vi "MT Generate PAM system parameters (M).vi"(0 "samples per symbol (16)":i32=16, 5 "M-PAM (2)":i32=2, 11 "error in (no error)":errorcluster) -> (6 "PAM system parameters":T1 {"symbol map" format="%.3f"}, 8 "bits per symbol":i32, 15 "error out":errorcluster)   [LabVIEW 2020, in "niDMT.lvlib"]
doc: "This polymorphic instance calculates parameters for use with either the MT Modulate PAM VI or the MT Demodulate PAM VI. It accepts an M-ary value that specifies a predefined symbol map with the number of distinct levels to use as symbols."
uses:
  <vilib>/addons/Modulation/niDMT.lvlib
  <vilib>/addons/Modulation/Digital/Support/Controls/PAM system parameters.ctl
  <vilib>/addons/Modulation/niAMT.lvlib
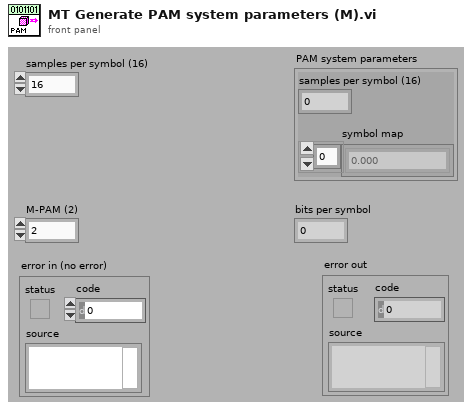
[diagram p1: front panel]
types:
  T1 = cluster{"samples per symbol (16)":i32, "symbol map":cdb[]}
  T2 = typedef "niDMT.lvlib/PAM system parameters.ctl" = cluster{"samples per symbol (16)":i32, "symbol map":cdb[]}
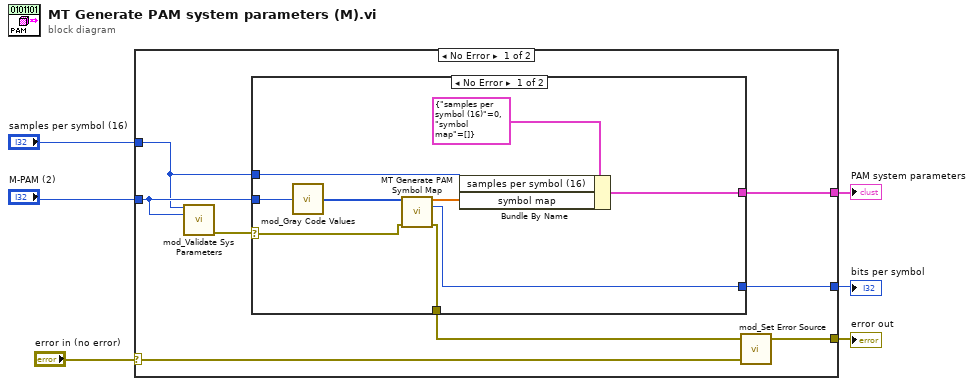
[diagram p0: block diagram]
diagram:
  n1 = case shown="No Error" "error in (no error)" {
    selector: "error in (no error)" -> [w10 w25]
    tunnel: "M-PAM (2)" -> [w9 _]
    tunnel: "samples per symbol (16)" -> [w8 _]
    tunnel: [w13 _] -> w4
    tunnel: [w12 _] -> w3
    tunnel: [w11 w25] -> w2
    frame No Error {
      n2 = call <vilib>:"mod_Validate Sys Parameters.vi"("samples per symbol"=w8, "M-ary"=w9) -> ("error out"=w7:errorcluster)  [unwired: 13 out]
      n3 = case shown="No Error" w7 {
        selector: w7 -> [w15 w24]
        tunnel: w9 -> [w23 _]
        tunnel: [w19 w24] -> w14
        tunnel: w8 -> [w18 _]
        tunnel: [w17 _] -> w13
        tunnel: [w16 _] -> w12
        frame No Error {
          n4 = call <vilib>:"mod_Gray Code Values.vi"("M"=w23) -> ("Gray coded values"=w22:i32[])
          n5 = call <vilib>:"MT Generate PAM Symbol Map.vi"("symbol values"=w22, "error in (no error)"=w15) -> ("symbol map"=w20:cdb[], "bits per symbol"=w16:i32, "error out"=w19:errorcluster)  [unwired: 11 out]
          n6 = Bundle By Name(cluster=T2 {"samples per symbol (16)"=0, "symbol map"=[]} ("PAM System Parameters"), "samples per symbol (16)"=w18, "symbol map"=w20) -> (w17:T2)
        }
        frame Error {
        }
      }
      n7 = call <vilib>:"mod_Set Error Source.vi"("initial error in (no error)"=w10, "final error in (no error)"=w14) -> ("error out"=w11:errorcluster)  [unwired: 3 out]
    }
    frame Error {
    }
  }
  "PAM system parameters" <- w4
  "bits per symbol" <- w3
  "error out" <- w2
